vi "Main.vi"() -> ()   [LabVIEW 2016]
uses:
  MainFGV/modes_mains_FGV.ctl
  Tools/three_modes.ctl
  Tools/control_modes.ctl
  Tools/control_data.ctl
  MainFGV/cluster_main_FGV.ctl
  Config/Channel_config.ctl
  Config/essay_config.ctl
  Tools/record_modes.ctl
  StepMotor/step_motor_modes.ctl
  <vilib>/ptbypt/NI_PtbyPt.lvlib
panel:
  out "StepAborted":bool
  out "FimFuro":bool
  in  "Comment":bool
  out "error out":errorcluster
  in  "NextStep":bool
  in  "ConfigStep":bool caption="Configurar ensaio"
  out "CurDep":dbl(slide) caption="Profundidade atual"
  in  "Avançar":bool
  in  "ContA":bool=TRUE caption="Controle automático"
  out "Graf":dbl[][](graph)
  in  "CP":bool caption="Cancelar ponto"
  in  "StartAuto":bool
  in  "Sim.":bool caption="Simulação"
  out "Log":string
  in  "NP":tag="PXI1Slot4_2" caption="Nome da placa"
  in  "NE":string caption="Nome do ensaio"
  in  "DE":path=path "C:/Users/l01481/Desktop/Teste" caption="Diretório do ensaio"
  out "G":u8(slide) caption="Gravação" scale=0.0..100.0
  in  "RP":bool caption="Registrar ponto"
  in  "Zerar":bool
  in  "PA":bool caption="Parar aquisição"
  in  "CC":bool caption="Configurar ensaio"
  in  "InitAcq":bool
  # "Programa de tensão residual - Aquisição"
  # "Configurações iniciais"
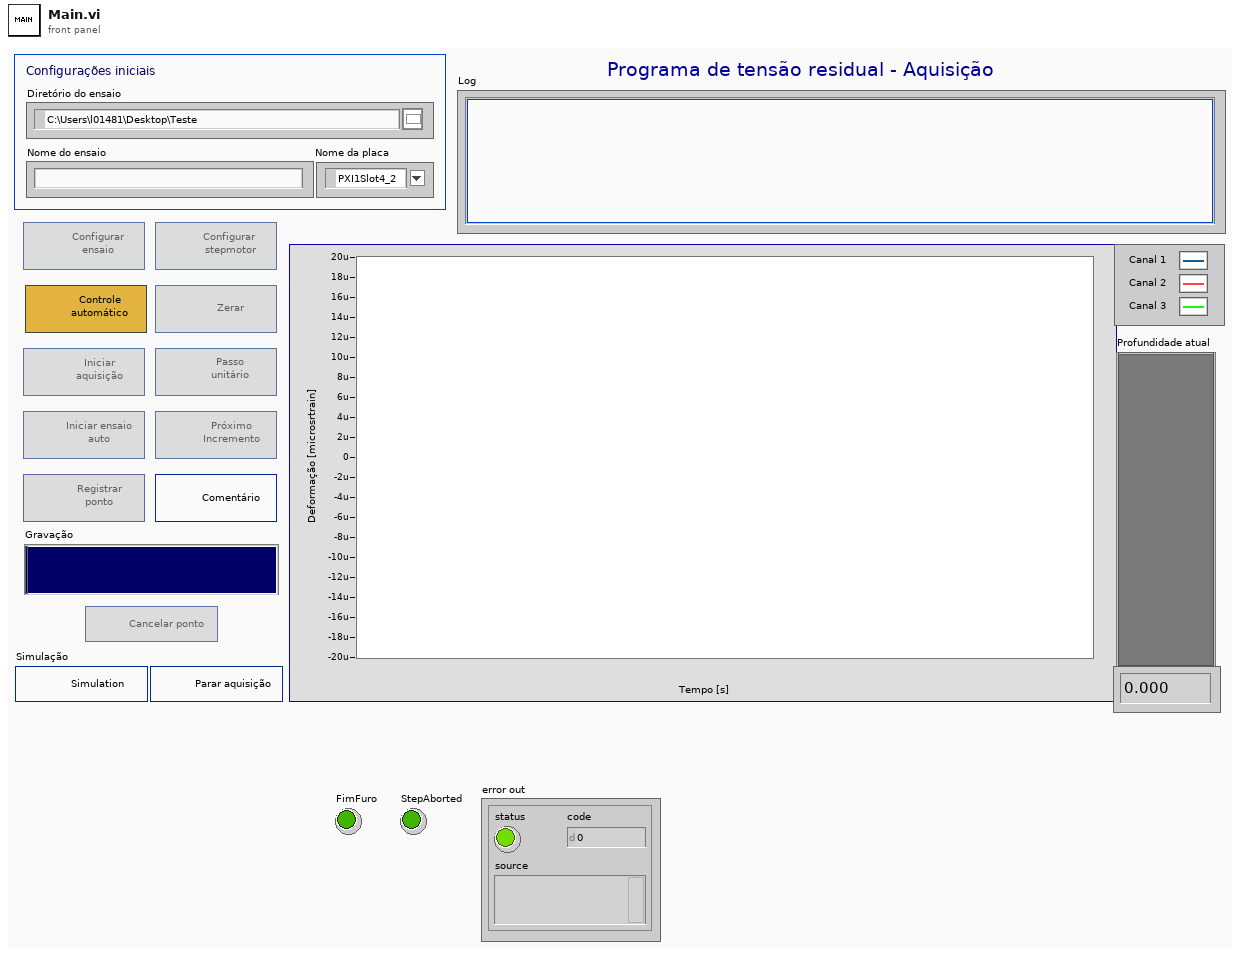
[diagram p1: front panel]
types:
  T1 = typedef "step_motor_modes.ctl" = enum16{"Init", "Config", "OpenCom", "Ajuste", "Step", "End"}
  T2 = typedef "modes_mains_FGV.ctl" = enum16{"Init", "Config", "CreateDir", "CreateTask", "CreateQueues", "Record", "Comment", "End"}
  T3 = typedef "record_modes.ctl" = enum16{"Grava vetor", "Acumula vetor", "Aguarda comando", "Cancela ponto"}
  T4 = typedef "control_modes.ctl" = enum16{"Concluir ensaio", "Calibrar", "Abortar", "Init", "Zerar", "Zero", "Canc. Pon.", "Esp. abertura", "Grava", "Esp. estab.", "EspFimFuro", "Cancelar"}
  T5 = typedef "cluster_main_FGV.ctl" = cluster{"Simulation?":bool, "ChanConfigs":T6[], "Essay Config":T7, "Directory":path, "EssayName":string, "RawFile":refnum<file>, "InfoFile":refnum<file>, "DataFile":refnum<file>, "task":refnum<k21>, "qRecord":refnum<queue>, "qProcess":refnum<queue>}
  T6 = typedef "Channel_config.ctl" = cluster{"Canal":i32, "GF":dbl, "SC":bool}
  T7 = typedef "essay_config.ctl" = cluster{"HoleDiam":dbl, "MeanLineDiam":dbl, "IncF":dbl, "ElastMod":dbl, "PoissonMod":dbl, "RosType":enum16{"Tipo A", "Tipo B", "Tipo C"}, "Método de análise":enum16{"Não uniforme 2013", "Simplificado 2013", "Simplificado 2008"}, "Pfinal":dbl, "AStop":bool}
  T8 = typedef "control_data.ctl" = cluster{"ContZ":i32, "ContAcimaZ":i32, "TentativasZ":i32, "Limiar DesvP":dbl, "ContCal":i32, "ContEstab":i32, "ContNEstab":i32, "ContGravando":i32, "ContParaVoltar":i32}
  T9 = typedef "three_modes.ctl" = enum16{"Init", "Exec", "End"}
  T10 = enum8{"Enabled", "Disabled", "Disabled and Grayed Out"}
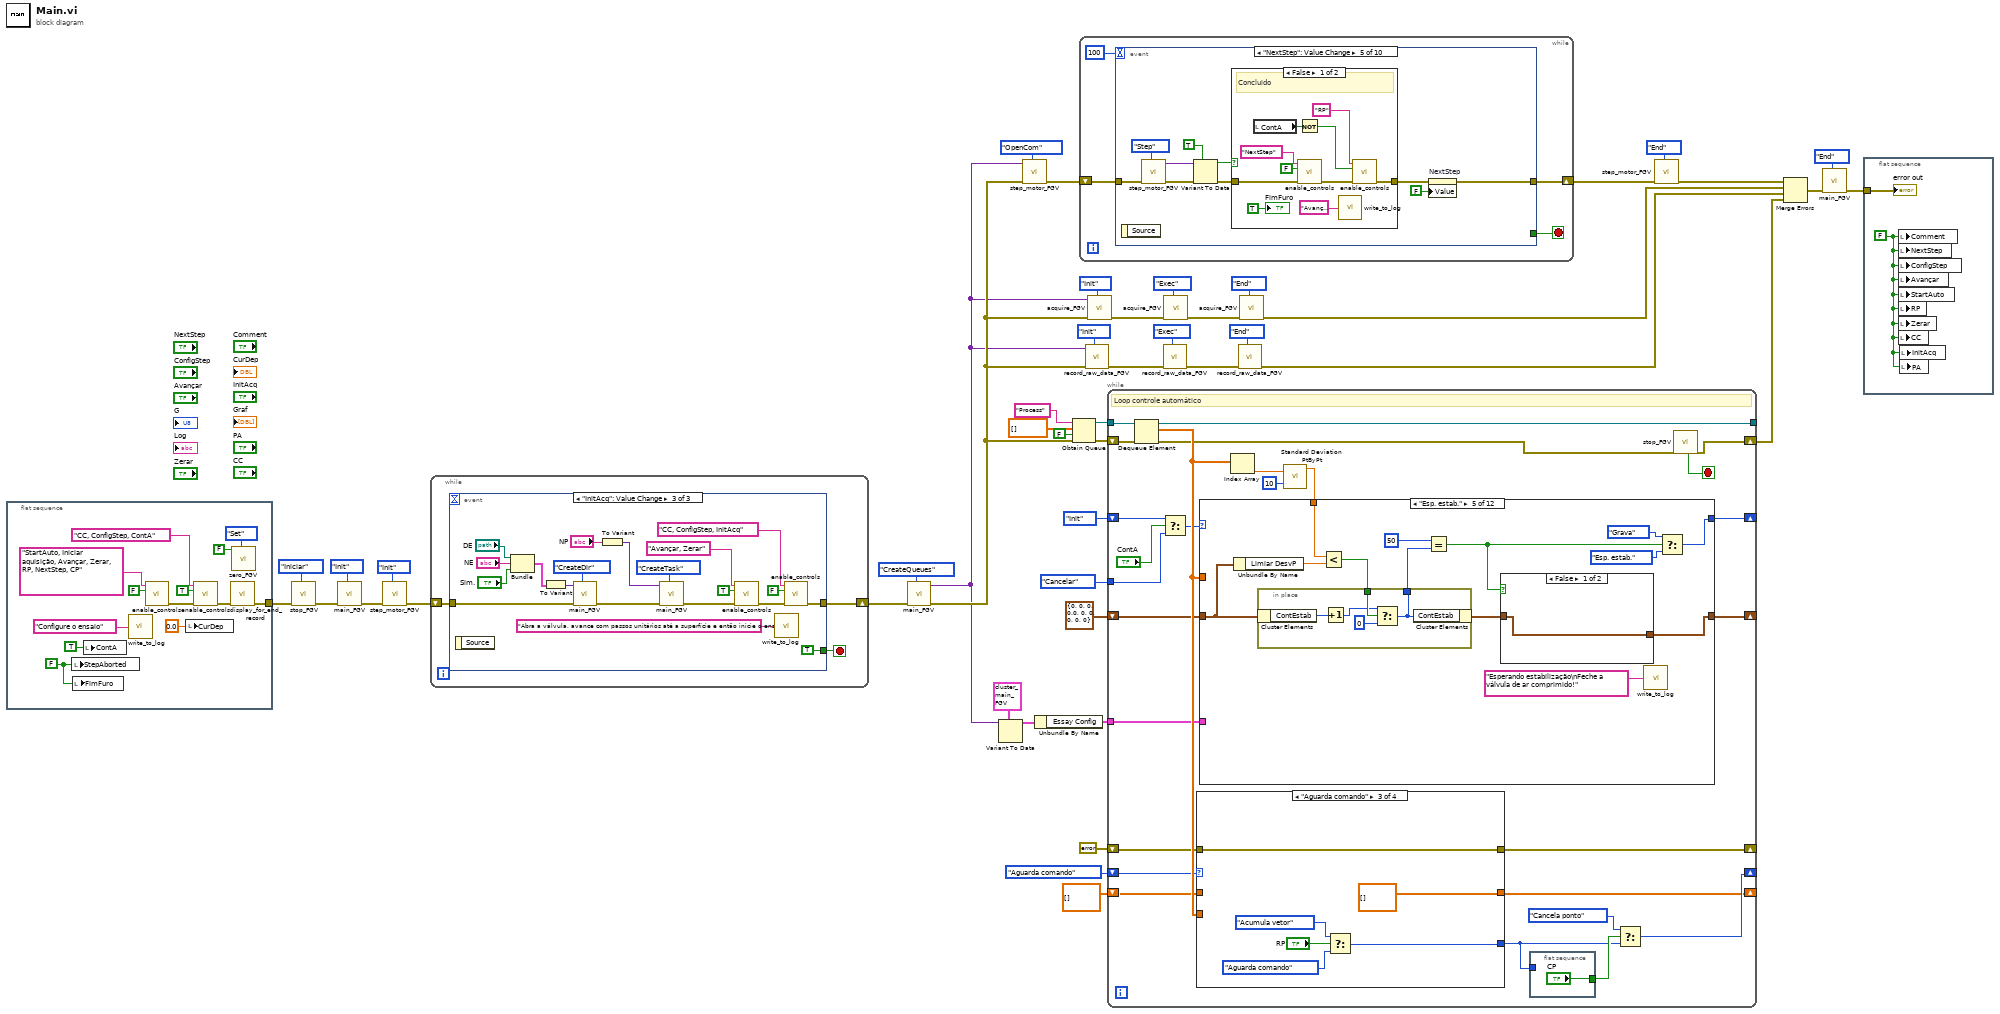
[diagram p0: block diagram]
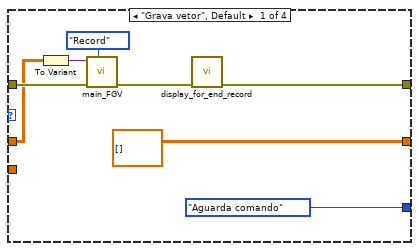
[diagram p2: hidden frame]
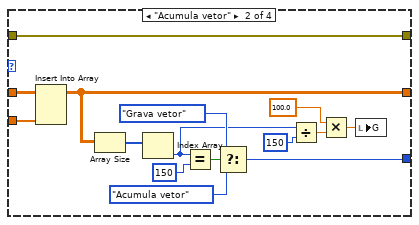
[diagram p3: hidden frame]
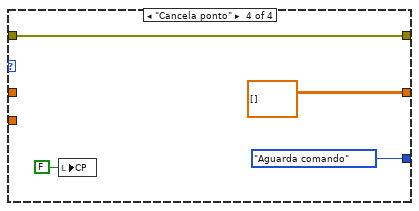
[diagram p4: hidden frame]
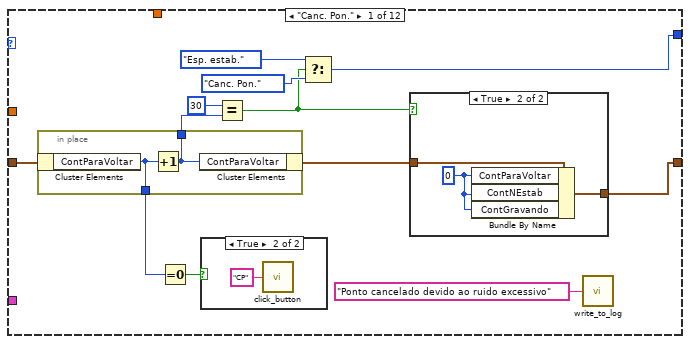
[diagram p5: hidden frame]
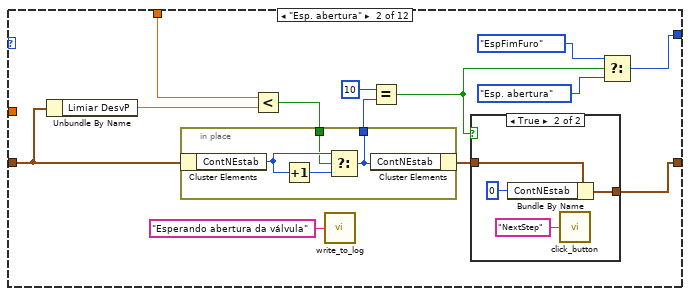
[diagram p8: hidden frame]
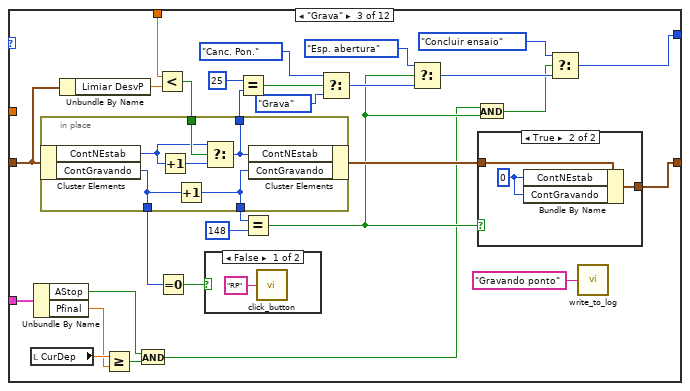
[diagram p10: hidden frame]
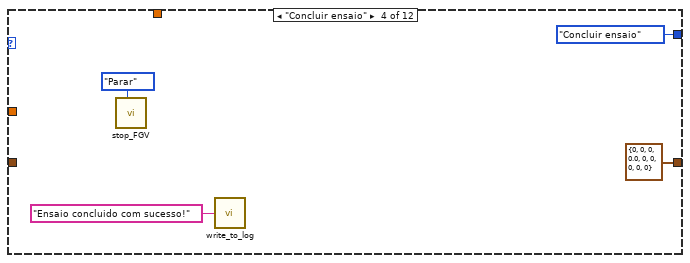
[diagram p13: hidden frame]
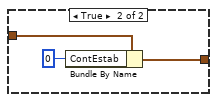
[diagram p14: hidden frame]
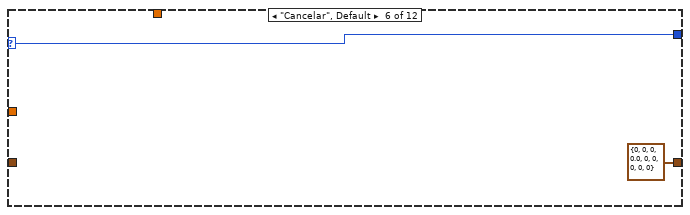
[diagram p15: hidden frame]
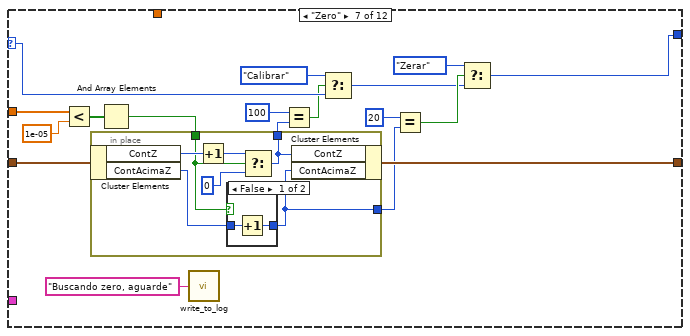
[diagram p16: hidden frame]
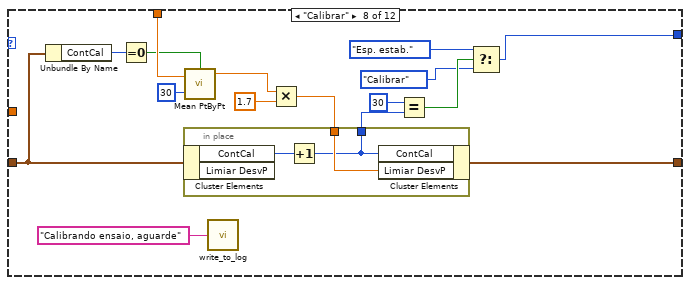
[diagram p18: hidden frame]
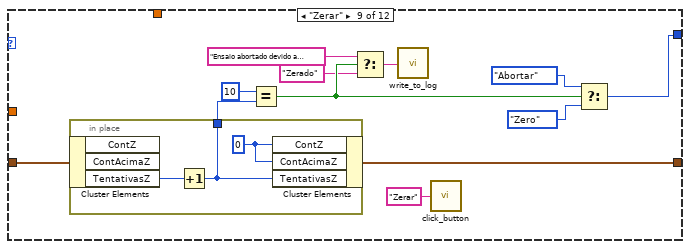
[diagram p19: hidden frame]
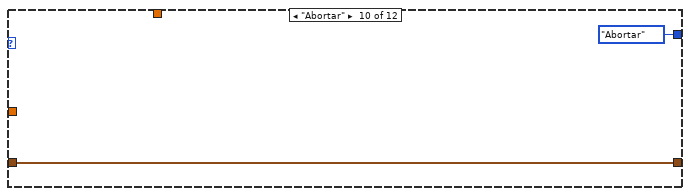
[diagram p20: hidden frame]
diagram:
  n1 = flat-sequence {
    tunnel: [w51] -> w3
    frame #0 {
      w47 = FALSE ("StepAborted")
      n2 = local write "StepAborted"(w47) -> ()
      n3 = local write "FimFuro"(w47) -> ()
      n4 = local write "ContA"(TRUE ("ContA")) -> ()
      n5 = call "write_to_log.vi"("Log"="Configure o ensaio") -> ()  [unwired: 5 in]
      n6 = call "enable_controls.vi"("Enable?"=FALSE, "Controls Label"="StartAuto, Iniciar aquisição, Avançar, Zerar, RP, NextStep, CP" ("name (unnamed)")) -> ("error out"=w55:errorcluster)  [unwired: 9 in]
      n7 = local write "CurDep"(0.0 ("CurDep")) -> ()
      n8 = call "enable_controls.vi"("error in"=w55, "Enable?"=TRUE, "Controls Label"="CC, ConfigStep, ContA" ("name (unnamed)")) -> ("error out"=w52:errorcluster)  [unwired: 8 in]
      n9 = call "display_for_end_record.vi"("error in"=w52) -> ("error out"=w51:errorcluster)  [unwired: 10 in]
      n10 = call "zero_FGV.vi"("comandos"=enum16{"Set", "Zerar?"}."Set", "Value"=FALSE) -> ()  [unwired: 9 in, 1 out]
    }
  }
  n11 = call "stop_FGV.vi"("comandos"=enum16{"Iniciar", "Parar", "Parar?"}."Iniciar", "error in (no error)"=w3) -> ("error out"=w2:errorcluster)  [unwired: 8 in, 1 out]
  n12 = call "main_FGV.vi"("Mode"=modes_mains_FGV."Init", "error in"=w2) -> ("error out"=w20:errorcluster)  [unwired: 8 in, 1 out]
  n13 = call "step_motor_FGV.vi"("Mode"=step_motor_modes."Init", "error in"=w20) -> ("error out"=w19:errorcluster)  [unwired: 8 in, 1 out]
  n14 = while {
    shift-right: [w61] -> w17
    shift-left: w19 -> [w62]
    stop <- w60 stop-if-true
    n15 = event shown="[2] \"InitAcq\": Value Change" {
      selector: _ -> [_ _ _]
      dyn-events: _ -> [_ _ _]
      timeout: _ -> [_ _ _]
      tunnel: w62 -> [w71 w76 w96]
      tunnel: [w66 w74 w80] -> w61
      tunnel: [_ _ TRUE] -> w60
      event "CC": Value Change {
        n16 = event-data() -> ()  [unwired: 1 in, 1 out]
        n17 = control-ref of="InitAcq"() -> (w69:refnum<vi>)
        n18 = call "main_FGV.vi"("Mode"=modes_mains_FGV."Config", "error in"=w71) -> ("error out"=w68:errorcluster)  [unwired: 8 in, 1 out]
        n19 = property class="Bool (strict)"(reference=w69, error in=w68, "DisabledEnum"=T10."Enabled" ("Disabled")) -> (error out=w67:errorcluster)  [unwired: 1 out]
        n20 = control-ref of="CC"() -> (w65:refnum<vi>)
        n21 = property class="Bool (strict)"(reference=w65, error in=w67, "Value"=FALSE) -> (error out=w66:errorcluster)  [unwired: 1 out]
        n22 = call "write_to_log.vi"("Log"="Inicie a aquisição") -> ()  [unwired: 5 in]
      }
      event "ConfigStep": Value Change {
        n23 = event-data() -> ()  [unwired: 1 in, 1 out]
        n24 = call "step_motor_FGV.vi"("Mode"=step_motor_modes."Config", "error in"=w76) -> ("error out"=w75:errorcluster)  [unwired: 8 in, 1 out]
        n25 = property on="ConfigStep" class="Bool (strict)"(error in=w75, "Value"=FALSE ("ConfigStep")) -> (error out=w74:errorcluster)  [unwired: 1 in, 1 out]
      }
      event "InitAcq": Value Change {
        n26 = event-data() -> ()  [unwired: 1 in, 1 out]
        n27 = Bundle("DE"="DE", "NE"="NE", "Sim."="Sim.") -> (w95:cluster{"DE":path, "NE":string, "Sim.":bool})  [unwired: 1 in]
        n28 = To Variant(anything=w95) -> (Variant=w92:variant)
        n29 = call "main_FGV.vi"("Mode"=modes_mains_FGV."CreateDir", "error in"=w96, "Parameter in"=w92) -> ("error out"=w90:errorcluster)  [unwired: 7 in, 1 out]
        n30 = To Variant(anything="NP") -> (Variant=w88:variant)
        n31 = call "main_FGV.vi"("Mode"=modes_mains_FGV."CreateTask", "error in"=w90, "Parameter in"=w88) -> ("error out"=w84:errorcluster)  [unwired: 7 in, 1 out]
        n32 = call "enable_controls.vi"("error in"=w84, "Enable?"=TRUE, "Controls Label"="Avançar, Zerar" ("name (unnamed)")) -> ("error out"=w81:errorcluster)  [unwired: 8 in]
        n33 = call "write_to_log.vi"("Log"="Abra a válvula, avance com passos unitários até a superfície e então inicie o ensaio automático") -> ()  [unwired: 5 in]
        n34 = call "enable_controls.vi"("error in"=w81, "Enable?"=FALSE, "Controls Label"="CC, ConfigStep, InitAcq" ("name (unnamed)")) -> ("error out"=w80:errorcluster)  [unwired: 8 in]
      }
    }
  }
  n35 = call "main_FGV.vi"("Mode"=modes_mains_FGV."CreateQueues", "error in"=w17) -> ("error out"=w16:errorcluster, "Parameter out"=w14:variant)  [unwired: 8 in]
  n36 = Variant To Data(type=T5 {"Simulation?"=FALSE, "ChanConfigs"=[], "Essay Config"={"HoleDiam"=1.4, "MeanLineDiam"=5.0, "IncF"=0.2, "ElastMod"=207.0, "PoissonMod"=0.3, "RosType"=enum."Tipo A", "Método de análise"=enum."Simplificado 2008", "Pfinal"=0.3, "AStop"=TRUE}, "Directory"=path "", "EssayName"="", "RawFile"=refnum, "InfoFile"=refnum, "DataFile"=refnum, "task"="", "qRecord"=refnum, "qProcess"=refnum} ("cluster_main_FGV"), Variant=w14) -> (data=w26:T5)  [unwired: 1 in, 1 out]
  n37 = call "step_motor_FGV.vi"("Mode"=step_motor_modes."OpenCom", "error in"=w16, "Parameter in"=w14) -> ("error out"=w15:errorcluster)  [unwired: 7 in, 1 out]
  n38 = Unbundle By Name(w26) -> ("Essay Config"=w25:T7)
  n39 = Obtain Queue(name (unnamed)="Process", element data type=dbl[] [] ("2D array"), create if not found? (T)=FALSE, error in (no error)=w16) -> (queue out=w30:refnum<queue>, error out=w31:errorcluster)  [unwired: 1 in, 1 out]
  n40 = while {
    shift-right: [w98] -> w10
    shift-left: w15 -> [w101]
    stop <- w99 stop-if-true
    n41 = event shown="[4] \"NextStep\": Value Change" {
      selector: _ -> [_ _ _ _ _ _ _ _ _ _]
      dyn-events: _ -> [_ _ _ _ _ _ _ _ _ _]
      timeout: 100 -> [_ _ _ _ _ _ _ _ _ _]
      tunnel: w101 -> [w105 w116 w120 w141 w153 w175 w181 w187 w192 w197]
      tunnel: [w102 w117 _ _ _ _ _ _ _ _] -> w99
      tunnel: [w104 w115 w123 w136 w146 w169 w176 w182 w191 w196] -> w98
      event "PA": Value Change {
        n42 = event-data() -> ()  [unwired: 1 in, 1 out]
        n43 = Two Button Dialog(message="Esta ação abortará o ensaio.\nDeseja continuar?", 1:"Cancelar" ("F button name (\"Cancel\")")) -> (T button?=w103:bool)  [unwired: 1 in]
        n44 = case shown="True" w103 {
          tunnel: w105 -> [w109 w112]
          tunnel: [w109 w111] -> w104
          tunnel: [FALSE ("parar?") w110] -> w102
          frame False {
          }
          frame True {
            n45 = call "stop_FGV.vi"("comandos"=enum16{"Iniciar", "Parar", "Parar?"}."Parar", "error in (no error)"=w112) -> ("error out"=w111:errorcluster, "parar?"=w110:bool)  [unwired: 8 in]
          }
        }
      }
      event Timeout {
        n46 = event-data() -> ()  [unwired: 1 in, 1 out]
        n47 = local read "ContA"() -> (w114:bool)
        n48 = case shown="True" w114 {
          frame False {
            n49 = call "write_to_log.vi"("Log"="Controle automático cancelado, conclua o ensaio manualmente") -> ()  [unwired: 5 in]
          }
          frame True {
          }
        }
        n50 = call "stop_FGV.vi"("error in (no error)"=w116) -> ("error out"=w115:errorcluster, "parar?"=w117:bool)  [unwired: 9 in]
      }
      event "Avançar": Value Change {
        n51 = event-data() -> ()  [unwired: 1 in, 1 out]
        n52 = First Call?() -> (First Call?: T/F=w121:bool)
        n53 = case shown="True" w121 {
          tunnel: w120 -> [w126 w129]
          tunnel: [w126 w128] -> w119
          frame False {
          }
          frame True {
            n54 = call "write_to_log.vi"("Log"="Certifique-se de fechar a válvula de ar comprimido antes de iniciar o ensaio automático" ("Controls Label")) -> ()  [unwired: 5 in]
            n55 = Two Button Dialog(message="Certifique-se que a válvula está aberta antes de avançar!", 1:"Cancelar" ("F button name (\"Cancel\")"), 2:"Avançar!" ("T button name (\"OK\")")) -> ()  [unwired: 1 out]
            n56 = call "enable_controls.vi"("error in"=w129, "Enable?"=TRUE, "Controls Label"="StartAuto") -> ("error out"=w128:errorcluster)  [unwired: 8 in]
          }
        }
        n57 = call "step_motor_FGV.vi"("Mode"=step_motor_modes."Ajuste", "error in"=w119) -> ("error out"=w124:errorcluster)  [unwired: 8 in, 1 out]
        n58 = property on="Avançar" class="Bool (strict)"(error in=w124, "Value"=FALSE ("Avançar")) -> (error out=w123:errorcluster)  [unwired: 1 in, 1 out]
      }
      event "ContA": Value Change {
        n59 = event-data() -> ()  [unwired: 1 in, 1 out]
        n60 = call "write_to_log.vi"("Log"="Controle automático cancelado, conclua o ensaio manualmente") -> ()  [unwired: 5 in]
        n61 = call "enable_controls.vi"("error in"=w141, "Enable?"=TRUE, "Controls Label"="RP, NextStep, CP, Avançar" ("name (unnamed)")) -> ("error out"=w138:errorcluster)  [unwired: 8 in]
        n62 = call "enable_controls.vi"("error in"=w138, "Enable?"=FALSE, "Controls Label"="ContA" ("name (unnamed)")) -> ("error out"=w137:errorcluster)  [unwired: 8 in]
        n63 = property on="StartAuto" class="Bool (strict)"(error in=w137, "Value"=TRUE ("StartAuto")) -> (error out=w136:errorcluster)  [unwired: 1 in, 1 out]
      }
      event "NextStep": Value Change {
        n64 = event-data() -> ()  [unwired: 1 in, 1 out]
        n65 = call "step_motor_FGV.vi"("Mode"=step_motor_modes."Step", "error in"=w153) -> ("error out"=w152:errorcluster, "Parameter out"=w148:variant)  [unwired: 8 in]
        n66 = Variant To Data(error in=w152, type=TRUE ("FimFuro"), Variant=w148) -> (data=w149:bool, error out=w151:errorcluster)
        n67 = case shown="False" w149 {
          tunnel: w151 -> [w160 w167]
          tunnel: [w158 w167] -> w147
          frame False {
            # "Concluido"
            n68 = local read "ContA"() -> (w156:bool)
            n69 = Not(x=w156) -> (.not. x?=w155:bool)
            n70 = call "enable_controls.vi"("error in"=w160, "Enable?"=FALSE, "Controls Label"="NextStep") -> ("error out"=w159:errorcluster)  [unwired: 8 in]
            n71 = call "write_to_log.vi"("Log"="Avanço concluido" ("name (unnamed)")) -> ()  [unwired: 5 in]
            n72 = call "enable_controls.vi"("error in"=w159, "Enable?"=w155, "Controls Label"="RP") -> ("error out"=w158:errorcluster)  [unwired: 8 in]
            "FimFuro" <- TRUE ("FimFuro")
          }
          frame True {
            # "Cancelado"
            n73 = call "write_to_log.vi"("Log"="Avanço cancelado" ("name (unnamed)")) -> ()  [unwired: 5 in]
            "StepAborted" <- TRUE ("StepAborted")
          }
        }
        n74 = property on="NextStep" class="Bool (strict)"(error in=w147, "Value"=FALSE ("NextStep")) -> (error out=w146:errorcluster)  [unwired: 1 in, 1 out]
      }
      event "Comment": Value Change {
        n75 = event-data() -> ()  [unwired: 1 in, 1 out]
        n76 = call "Janela de comentário"("error in (no error)"=w175) -> ("Comentário"=w172:string, "error out"=w173:errorcluster)  [unwired: 16 in, 1 out]
        n77 = To Variant(anything=w172) -> (Variant=w171:variant)
        n78 = call "main_FGV.vi"("Mode"=modes_mains_FGV."Comment", "error in"=w173, "Parameter in"=w171) -> ("error out"=w170:errorcluster)  [unwired: 7 in, 1 out]
        n79 = property on="Comment" class="Bool (strict)"(error in=w170, "Value"=FALSE ("Comment")) -> (error out=w169:errorcluster)  [unwired: 1 in, 1 out]
      }
      event "RP": Value Change {
        w179 = TRUE ("Visible")
        n80 = event-data() -> ()  [unwired: 1 in, 1 out]
        n81 = property on="G" class="Slide (strict)"(error in=w181, "Visible"=w179) -> (error out=w180:errorcluster)  [unwired: 1 in, 1 out]
        n82 = property on="CP" class="Bool (strict)"(error in=w180, "Visible"=w179) -> (error out=w177:errorcluster)  [unwired: 1 in, 1 out]
        n83 = property on="RP" class="Bool (strict)"(error in=w177, "DisabledEnum"=T10."Disabled and Grayed Out" ("Disabled")) -> (error out=w176:errorcluster)  [unwired: 1 in, 1 out]
      }
      event "CP": Value Change {
        n84 = event-data() -> ()  [unwired: 1 in, 1 out]
        n85 = call "display_for_end_record.vi"("error in"=w187) -> ("error out"=w183:errorcluster)  [unwired: 10 in]
        n86 = local read "ContA"() -> (w186:bool)
        n87 = Not(x=w186) -> (.not. x?=w185:bool)
        n88 = call "enable_controls.vi"("error in"=w183, "Enable?"=w185, "Controls Label"="RP") -> ("error out"=w182:errorcluster)  [unwired: 8 in]
      }
      event "StartAuto": Value Change {
        n89 = event-data() -> ()  [unwired: 1 in, 1 out]
        n90 = call "enable_controls.vi"("error in"=w192, "Enable?"=FALSE, "Controls Label"="Zerar, Avançar, StartAuto" ("name (unnamed)")) -> ("error out"=w191:errorcluster)  [unwired: 8 in]
        n91 = One Button Dialog(message="Feche a válvula de ar comprimido para que\n seja possível fazer a calibração do ensaio") -> ()  [unwired: 1 in, 1 out]
      }
      event "Zerar": Value Change {
        n92 = event-data() -> ()  [unwired: 1 in, 1 out]
        n93 = call "zero_FGV.vi"("comandos"=enum16{"Set", "Zerar?"}."Set", "Value"=TRUE) -> ("Zerar?"=w194:bool)  [unwired: 9 in]
        n94 = flat-sequence {
          tunnel: [dbl[][] [] ("History Data")] -> w195
          tunnel: w194 -> [_]
          tunnel: [FALSE ("Value")] -> w193
          frame #0 {
            n95 = Wait (ms)(milliseconds to wait=u32 150) -> ()  [unwired: 1 out]
          }
        }
        n96 = local write "Zerar"(w193) -> ()
        n97 = property on="Graf" class="WFChart (strict)"(error in=w197, "History Data"=w195) -> (error out=w196:errorcluster)  [unwired: 1 in, 1 out]
      }
    }
  }
  n98 = call "record_raw_data_FGV.vi"("Mode"=three_modes."Init", "error in"=w16, "Parameter in"=w14) -> ("error out"=w36:errorcluster)  [unwired: 7 in, 1 out]
  n99 = call "acquire_FGV.vi"("Mode"=three_modes."Init", "error in"=w16, "Parameter in"=w14) -> ("error out"=w41:errorcluster)  [unwired: 7 in, 1 out]
  n100 = while {
    shift-right: [w225] -> _
    shift-left: control_modes."Init" ("Enum") -> [w216]
    tunnel: w30 -> [w228]
    shift-right: [w217] -> w9
    shift-left: w31 -> [w227]
    tunnel: [w226] -> _
    shift-right: [w223] -> _
    shift-left: T8 {"ContZ"=0, "ContAcimaZ"=0, "TentativasZ"=0, "Limiar DesvP"=0.0, "ContCal"=0, "ContEstab"=0, "ContNEstab"=0, "ContGravando"=0, "ContParaVoltar"=0} ("Dados controlador") -> [w224]
    tunnel: w25 -> [w222]
    tunnel: control_modes."Cancelar" ("f") -> [w213]
    shift-right: [w208] -> _
    shift-left: record_modes."Aguarda comando" ("Estados") -> [w205]
    shift-right: [w207] -> _
    shift-left: dbl[][] [] -> [w206]
    shift-right: [w204] -> _
    shift-left: errorcluster {"status"=FALSE, "code"=0, "source"=""} ("error out") -> [w203]
    stop <- w212 stop-if-true
    # "Loop controle automático"
    n101 = Dequeue Element(queue=w228, error in (no error)=w227) -> (queue out=w226:refnum<queue>, element=w229:dbl[], error out=w218:errorcluster)  [unwired: 1 in, 1 out]
    n102 = Select(t=w216, s="ContA", f=w213) -> (s? t:f=w214:T4)
    n103 = case shown="\"Aguarda comando\"" w205 {
      tunnel: w229 -> [_ w253 _ _]
      tunnel: [record_modes."Aguarda comando" ("Estados") w245 w257 record_modes."Aguarda comando" ("Estados")] -> w209
      tunnel: [dbl[][] [] w251 dbl[][] [] dbl[][] []] -> w207
      tunnel: w206 -> [w232 w252 _ _]
      tunnel: [w236 w239 w255 w261] -> w204
      tunnel: w203 -> [w234 w239 w255 w261]
      frame "Grava vetor", Default {
        n104 = To Variant(anything=w232) -> (Variant=w231:variant)
        n105 = call "main_FGV.vi"("Mode"=modes_mains_FGV."Record", "error in"=w234, "Parameter in"=w231) -> ("error out"=w233:errorcluster)  [unwired: 7 in, 1 out]
        n106 = call "display_for_end_record.vi"("error in"=w233) -> ("error out"=w236:errorcluster)  [unwired: 10 in]
      }
      frame "Acumula vetor" {
        n107 = Insert Into Array(array=w252, new element=w253) -> (w251:dbl[][])  [unwired: 2 in]
        n108 = Array Size(array=w251) -> (size(s)=w250:i32[])
        n109 = Index Array(array=w250) -> (element=w244:i32)  [unwired: 1 in]
        n110 = Equal?(x=w244, y=150) -> (x = y?=w246:bool)
        n111 = Select(t=record_modes."Grava vetor" ("Estados"), s=w246, f=record_modes."Acumula vetor" ("Estados")) -> (s? t:f=w245:T3)
        n112 = Divide(x=w244, y=150) -> (x/y=w242:dbl)
        n113 = Multiply(x=100.0, y=w242) -> (x*y=w240:dbl)
        n114 = local write "G"(w240) -> ()
      }
      frame "Aguarda comando" {
        n115 = Select(t=record_modes."Acumula vetor" ("Estados"), s="RP", f=record_modes."Aguarda comando" ("Estados")) -> (s? t:f=w257:T3)
      }
      frame "Cancela ponto" {
        n116 = local write "CP"(FALSE ("CP")) -> ()
      }
    }
    n117 = Index Array(array=w229) -> (element=w220:dbl)  [unwired: 1 in]
    n118 = call <vilib>:"Standard Deviation PtByPt.vi"("x"=w220, "sample length"=10) -> ("standard deviation"=w219:dbl)  [unwired: 1 in, 2 out]
    n119 = case shown="\"Esp. estab.\"" w214 {
      selector: w214 -> [_ _ _ _ _ w372 w382 _ _ _ w441 _]
      tunnel: [w268 w287 w311 control_modes."Concluir ensaio" ("Enum") w356 w372 w374 w409 w425 control_modes."Abortar" ("Enum") w440 w451] -> w225
      tunnel: w224 -> [w275 w294 w332 _ w361 _ w388 w407 w431 w436 _ w443]
      tunnel: w229 -> [_ _ _ _ _ _ w390 _ _ _ _ _]
      tunnel: [w265 w288 w321 T8 {"ContZ"=0, "ContAcimaZ"=0, "TentativasZ"=0, "Limiar DesvP"=0.0, "ContCal"=0, "ContEstab"=0, "ContNEstab"=0, "ContGravando"=0, "ContParaVoltar"=0} ("Cluster") w351 T8 {"ContZ"=0, "ContAcimaZ"=0, "TentativasZ"=0, "Limiar DesvP"=0.0, "ContCal"=0, "ContEstab"=0, "ContNEstab"=0, "ContGravando"=0, "ContParaVoltar"=0} ("Cluster") w385 w415 w428 w436 T8 {"ContZ"=0, "ContAcimaZ"=0, "TentativasZ"=0, "Limiar DesvP"=0.0, "ContCal"=0, "ContEstab"=0, "ContNEstab"=0, "ContGravando"=0, "ContParaVoltar"=0} ("Cluster") w442] -> w223
      tunnel: w222 -> [_ _ w317 _ _ _ _ _ _ _ _ _]
      tunnel: w219 -> [_ w286 w318 _ w350 _ _ w408 _ _ _ _]
      frame "Canc. Pon." {
        n120 = in-place {
          in-place-border: [w282] -> w274
          in-place-border: [w281] -> w272
          n121 = in-place-cluster #1(w275) -> ("ContParaVoltar"=w282:i32)
          n122 = Increment(x=w282) -> (x+1=w281:i32)
          n123 = in-place-cluster #1("ContParaVoltar"=w281) -> (w266:T8)
        }
        n124 = Equal To 0?(x=w274) -> (x = 0?=w273:bool)
        n125 = case shown="True" w273 {
          frame False {
          }
          frame True {
            n126 = call "click_button.vi"("ButtonLabel"="CP") -> ()  [unwired: 5 in]
          }
        }
        n127 = Equal?(x=30, y=w272) -> (x = y?=w267:bool)
        n128 = Select(t=control_modes."Esp. estab." ("Enum"), s=w267, f=control_modes."Canc. Pon." ("Enum")) -> (s? t:f=w268:T4)
        n129 = case shown="True" w267 {
          tunnel: w266 -> [w276 w279]
          tunnel: [w276 w278] -> w265
          frame False {
          }
          frame True {
            w277 = 0 ("ContParaVoltar")
            n130 = Bundle By Name(cluster=w279, "ContParaVoltar"=w277, "ContNEstab"=w277, "ContGravando"=w277) -> (w278:T8)
          }
        }
        n131 = call "write_to_log.vi"("Log"="Ponto cancelado devido ao ruido excessivo") -> ()  [unwired: 5 in]
      }
      frame "Esp. abertura" {
        n132 = Unbundle By Name(w294) -> ("Limiar DesvP"=w295:dbl)
        n133 = Less?(x=w286, y=w295) -> (x < y?=w285:bool)
        n134 = in-place {
          in-place-border: w285 -> [w302]
          in-place-border: [w301] -> w293
          n135 = in-place-cluster #2(w294) -> ("ContNEstab"=w303:i32)
          n136 = Increment(x=w303) -> (x+1=w304:i32)
          n137 = Select(t=w303, s=w302, f=w304) -> (s? t:f=w301:i32)
          n138 = in-place-cluster #2("ContNEstab"=w301) -> (w289:T8)
        }
        n139 = call "write_to_log.vi"("Log"="Esperando abertura da válvula") -> ()  [unwired: 5 in]
        n140 = Equal?(x=10, y=w293) -> (x = y?=w290:bool)
        n141 = case shown="True" w290 {
          tunnel: w289 -> [w296 w300]
          tunnel: [w296 w298] -> w288
          frame False {
          }
          frame True {
            n142 = Bundle By Name(cluster=w300, "ContNEstab"=0) -> (w298:T8)
            n143 = call "click_button.vi"("ButtonLabel"="NextStep") -> ()  [unwired: 5 in]
          }
        }
        n144 = Select(t=control_modes."EspFimFuro" ("Enum"), s=w290, f=control_modes."Esp. abertura" ("Enum")) -> (s? t:f=w287:T4)
      }
      frame "Grava" {
        n145 = local read "CurDep"() -> (w316:dbl)
        n146 = Unbundle By Name(w317) -> ("AStop"=w313:bool, "Pfinal"=w315:dbl)
        n147 = Unbundle By Name(w332) -> ("Limiar DesvP"=w333:dbl)
        n148 = Greater Or Equal?(x=w316, y=w315) -> (x >= y?=w314:bool)
        n149 = And(x=w313, y=w314) -> (x .and. y?=w308:bool)
        n150 = Less?(x=w318, y=w333) -> (x < y?=w331:bool)
        n151 = in-place {
          in-place-border: w331 -> [w343]
          in-place-border: [w340] -> w330
          in-place-border: [w339] -> w327
          in-place-border: [w338] -> w320
          n152 = in-place-cluster #3(w332) -> ("ContNEstab"=w342:i32, "ContGravando"=w338:i32)
          n153 = Increment(x=w342) -> (x+1=w341:i32)
          n154 = Increment(x=w338) -> (x+1=w339:i32)
          n155 = Select(t=w342, s=w343, f=w341) -> (s? t:f=w340:i32)
          n156 = in-place-cluster #3("ContNEstab"=w340, "ContGravando"=w339) -> (w322:T8)
        }
        n157 = Equal To 0?(x=w320) -> (x = 0?=w319:bool)
        n158 = case shown="False" w319 {
          frame False {
            n159 = call "click_button.vi"("ButtonLabel"="RP") -> ()  [unwired: 5 in]
          }
          frame True {
          }
        }
        n160 = Equal?(x=25, y=w330) -> (x = y?=w326:bool)
        n161 = Equal?(x=w327, y=148 ("x")) -> (x = y?=w309:bool)
        n162 = Select(t=control_modes."Canc. Pon." ("Enum"), s=w326, f=control_modes."Grava" ("Enum")) -> (s? t:f=w323:T4)
        n163 = Select(t=control_modes."Esp. abertura" ("Enum"), s=w309, f=w323) -> (s? t:f=w312:T4)
        n164 = And(x=w308, y=w309) -> (x .and. y?=w307:bool)
        n165 = case shown="True" w309 {
          tunnel: w322 -> [w334 w337]
          tunnel: [w334 w336] -> w321
          frame False {
          }
          frame True {
            w335 = 0 ("ContNEstab")
            n166 = Bundle By Name(cluster=w337, "ContNEstab"=w335, "ContGravando"=w335) -> (w336:T8)
          }
        }
        n167 = Select(t=control_modes."Concluir ensaio" ("Enum"), s=w307, f=w312) -> (s? t:f=w311:T4)
        n168 = call "write_to_log.vi"("Log"="Gravando ponto") -> ()  [unwired: 5 in]
      }
      frame "Concluir ensaio" {
        n169 = call "stop_FGV.vi"("comandos"=enum16{"Iniciar", "Parar", "Parar?"}."Parar") -> ()  [unwired: 9 in, 2 out]
        n170 = call "write_to_log.vi"("Log"="Ensaio concluido com sucesso!") -> ()  [unwired: 5 in]
      }
      frame "Esp. estab." {
        n171 = Unbundle By Name(w361) -> ("Limiar DesvP"=w360:dbl)
        n172 = Less?(x=w350, y=w360) -> (x < y?=w359:bool)
        n173 = in-place {
          in-place-border: w359 -> [w370]
          in-place-border: [w366] -> w358
          n174 = in-place-cluster #4(w361) -> ("ContEstab"=w369:i32)
          n175 = Increment(x=w369) -> (x+1=w368:i32)
          n176 = Select(t=w368, s=w370, f=0) -> (s? t:f=w366:i32)
          n177 = in-place-cluster #4("ContEstab"=w366) -> (w353:T8)
        }
        n178 = Equal?(x=50, y=w358) -> (x = y?=w352:bool)
        n179 = case shown="False" w352 {
          tunnel: w353 -> [w362 w365]
          tunnel: [w362 w363] -> w351
          frame False {
          }
          frame True {
            n180 = Bundle By Name(cluster=w365, "ContEstab"=0 ("ContZ")) -> (w363:T8)
          }
        }
        n181 = call "write_to_log.vi"("Log"="Esperando estabilização\nFeche a válvula de ar comprimido!") -> ()  [unwired: 5 in]
        n182 = Select(t=control_modes."Grava" ("Enum"), s=w352, f=control_modes."Esp. estab." ("Enum")) -> (s? t:f=w356:T4)
      }
      frame "Cancelar", Default {
      }
      frame "Zero" {
        n183 = Less?(x=w390, y=1e-05) -> (x < y?=w387:bool[])
        n184 = And Array Elements(Boolean array=w387) -> (logical AND=w386:bool)
        n185 = in-place {
          in-place-border: w386 -> [w391]
          in-place-border: [w393] -> w384
          in-place-border: [w392] -> w379
          n186 = in-place-cluster #5(w388) -> ("ContZ"=w397:i32, "ContAcimaZ"=w394:i32)
          n187 = Increment(x=w397) -> (x+1=w396:i32)
          n188 = case shown="False" w391 {
            tunnel: w394 -> [w399 w400]
            tunnel: [w398 w400] -> w392
            frame False {
              n189 = Increment(x=w399) -> (x+1=w398:i32)
            }
            frame True {
            }
          }
          n190 = Select(t=w396, s=w391, f=0) -> (s? t:f=w393:i32)
          n191 = in-place-cluster #5("ContZ"=w393, "ContAcimaZ"=w392) -> (w385:T8)
        }
        n192 = call "write_to_log.vi"("Log"="Buscando zero, aguarde") -> ()  [unwired: 5 in]
        n193 = Equal?(x=100, y=w384) -> (x = y?=w380:bool)
        n194 = Select(t=control_modes."Calibrar", s=w380, f=w382) -> (s? t:f=w376:T4)
        n195 = Equal?(x=20, y=w379) -> (x = y?=w377:bool)
        n196 = Select(t=control_modes."Zerar", s=w377, f=w376) -> (s? t:f=w374:T4)
      }
      frame "Calibrar" {
        n197 = Unbundle By Name(w407) -> ("ContCal"=w406:i32)
        n198 = Equal To 0?(x=w406) -> (x = 0?=w405:bool)
        n199 = call <vilib>:"Mean PtByPt.vi"("x"=w408, "sample length"=30, "initialize"=w405) -> ("mean"=w404:dbl)  [unwired: 1 in, 1 out]
        n200 = call "write_to_log.vi"("Log"="Calibrando ensaio, aguarde") -> ()  [unwired: 5 in]
        n201 = Multiply(x=w404, y=1.7) -> (x*y=w402:dbl)
        n202 = in-place {
          in-place-border: w402 -> [w418]
          in-place-border: [w417] -> w414
          n203 = in-place-cluster #6(w407) -> ("ContCal"=w419:i32)  [unwired: 1 out]
          n204 = Increment(x=w419) -> (x+1=w417:i32)
          n205 = in-place-cluster #6("ContCal"=w417, "Limiar DesvP"=w418) -> (w415:T8)
        }
        n206 = Equal?(x=30, y=w414) -> (x = y?=w412:bool)
        n207 = Select(t=control_modes."Esp. estab." ("Enum"), s=w412, f=control_modes."Calibrar" ("Enum")) -> (s? t:f=w409:T4)
      }
      frame "Zerar" {
        n208 = in-place {
          in-place-border: [w432] -> w430
          w434 = 0 ("ContZ")
          n209 = in-place-cluster #7(w431) -> ("TentativasZ"=w433:i32)  [unwired: 2 out]
          n210 = Increment(x=w433) -> (x+1=w432:i32)
          n211 = in-place-cluster #7("ContZ"=w434, "ContAcimaZ"=w434, "TentativasZ"=w432) -> (w428:T8)
        }
        n212 = Equal?(x=10, y=w430) -> (x = y?=w424:bool)
        n213 = Select(t="Ensaio abortado devido a oscilação excessiva do sinal" ("Log"), s=w424, f="Zerado" ("Log")) -> (s? t:f=w420:string)
        n214 = call "write_to_log.vi"("Log"=w420) -> ()  [unwired: 5 in]
        n215 = call "click_button.vi"("ButtonLabel"="Zerar") -> ()  [unwired: 5 in]
        n216 = Select(t=control_modes."Abortar" ("Enum"), s=w424, f=control_modes."Zero" ("Enum")) -> (s? t:f=w425:T4)
      }
      frame "Abortar" {
      }
      frame "Init" {
        n217 = Select(t=control_modes."Zero", s="StartAuto", f=w441) -> (s? t:f=w440:T4)
      }
      frame "EspFimFuro" {
        n218 = local read "CurDep"() -> (w444:dbl)
        n219 = local read "FimFuro"() -> (w454:bool)
        n220 = Number To Fractional String(number=w444, precision (6)=i16 3) -> (F-format string=w448:string)  [unwired: 2 in]
        n221 = case shown="True" w454 {
          frame False {
          }
          frame True {
            n222 = local write "FimFuro"(FALSE ("FimFuro")) -> ()
          }
        }
        n223 = Select(t=control_modes."Esp. estab." ("Enum"), s=w454, f=control_modes."EspFimFuro" ("Enum")) -> (s? t:f=w453:T4)
        n224 = Concatenate Strings("Avançando até " ("string"), w448, " mm" ("string")) -> (w445:string)
        n225 = local read "StepAborted"() -> (w450:bool)
        n226 = call "write_to_log.vi"("Log"=w445) -> ()  [unwired: 5 in]
        n227 = Select(t=control_modes."Esp. abertura" ("f"), s=w450, f=w453) -> (s? t:f=w451:T4)
        n228 = case shown="True" w450 {
          tunnel: w443 -> [w457 w459]
          tunnel: [w457 w458] -> w442
          frame False {
          }
          frame True {
            n229 = in-place {
              n230 = in-place-cluster #8(w459) -> ()  [unwired: 1 out]
              n231 = in-place-cluster #8("ContNEstab"=-40) -> (w458:T8)
            }
            n232 = local write "StepAborted"(FALSE ("FimFuro")) -> ()
          }
        }
      }
    }
    n233 = flat-sequence {
      tunnel: ["CP"] -> w210
      tunnel: w209 -> [_]
      frame #0 {
      }
    }
    n234 = Select(t=record_modes."Cancela ponto" ("Estados"), s=w210, f=w209) -> (s? t:f=w208:T3)
    n235 = call "stop_FGV.vi"("error in (no error)"=w218) -> ("error out"=w217:errorcluster, "parar?"=w212:bool)  [unwired: 9 in]
  }
  n236 = call "record_raw_data_FGV.vi"("Mode"=three_modes."Exec", "error in"=w36) -> ("error out"=w35:errorcluster)  [unwired: 8 in, 1 out]
  n237 = call "acquire_FGV.vi"("Mode"=three_modes."Exec", "error in"=w41) -> ("error out"=w40:errorcluster)  [unwired: 8 in, 1 out]
  n238 = call "record_raw_data_FGV.vi"("Mode"=three_modes."End", "error in"=w35) -> ("error out"=w6:errorcluster)  [unwired: 8 in, 1 out]
  n239 = call "acquire_FGV.vi"("Mode"=three_modes."End", "error in"=w40) -> ("error out"=w7:errorcluster)  [unwired: 8 in, 1 out]
  n240 = call "step_motor_FGV.vi"("Mode"=step_motor_modes."End", "error in"=w10) -> ("error out"=w8:errorcluster)  [unwired: 8 in, 1 out]
  n241 = Merge Errors(w8, w7, w6, w9) -> (w5:errorcluster)
  n242 = call "main_FGV.vi"("Mode"=modes_mains_FGV."End", "error in"=w5) -> ("error out"=w4:errorcluster)  [unwired: 8 in, 1 out]
  n243 = flat-sequence {
    tunnel: w4 -> [w464]
    frame #0 {
      w463 = FALSE ("Comment")
      n244 = local write "Comment"(w463) -> ()
      n245 = local write "NextStep"(w463) -> ()
      n246 = local write "ConfigStep"(w463) -> ()
      n247 = local write "Avançar"(w463) -> ()
      n248 = local write "StartAuto"(w463) -> ()
      n249 = local write "RP"(w463) -> ()
      n250 = local write "Zerar"(w463) -> ()
      n251 = local write "CC"(w463) -> ()
      n252 = local write "InitAcq"(w463) -> ()
      n253 = local write "PA"(w463) -> ()
      "error out" <- w464
    }
  }
